vi "Tiepie-Initialize-2018-04-26.vi"(3 "error in (no error)":errorcluster, 4 "Sample Frequency/Hz":i32=500000000, 5 "Record Length/Samples":u64=50000, 6 "TiepieID":i32=33474) -> (0 "error out":errorcluster, 1 "TpDeviceHandle_t":u32, 2 "Card-OK":bool)   [LabVIEW 2013]
panel:
  in  "Channel 1_Range":dbl(ring)=0.4 items=["80 V"=80.0, "40 V"=40.0, "20 V"=20.0, "8 V"=8.0, "4 V"=4.0, "2 V"=2.0, "800 mV"=0.8, "400 mV"=0.4, "200 mV"=0.2]
  in  "CH1_Coupling":u64(ring)=1 items=["Volt DC"=1, "Volt AC"=2, "Ampere DC"=4, "Ampere AC"=8, "Ohm"=16]
  out "channelCount":u16
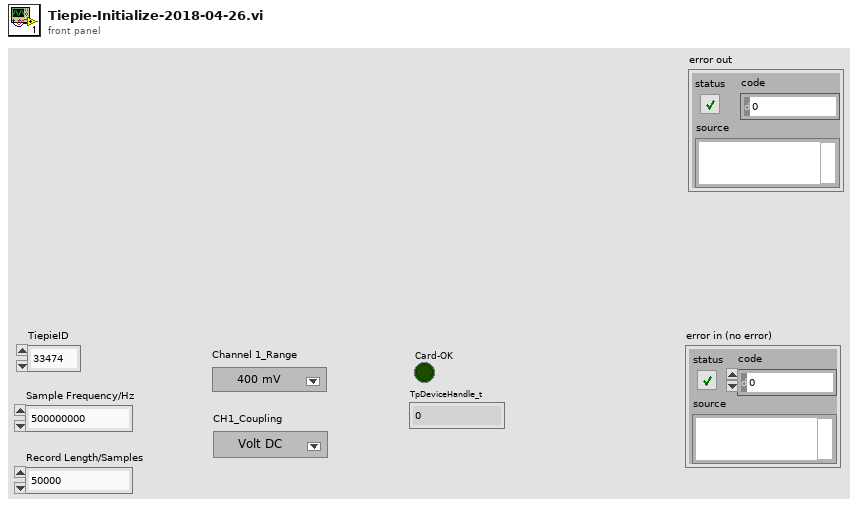
[diagram p1: front panel]
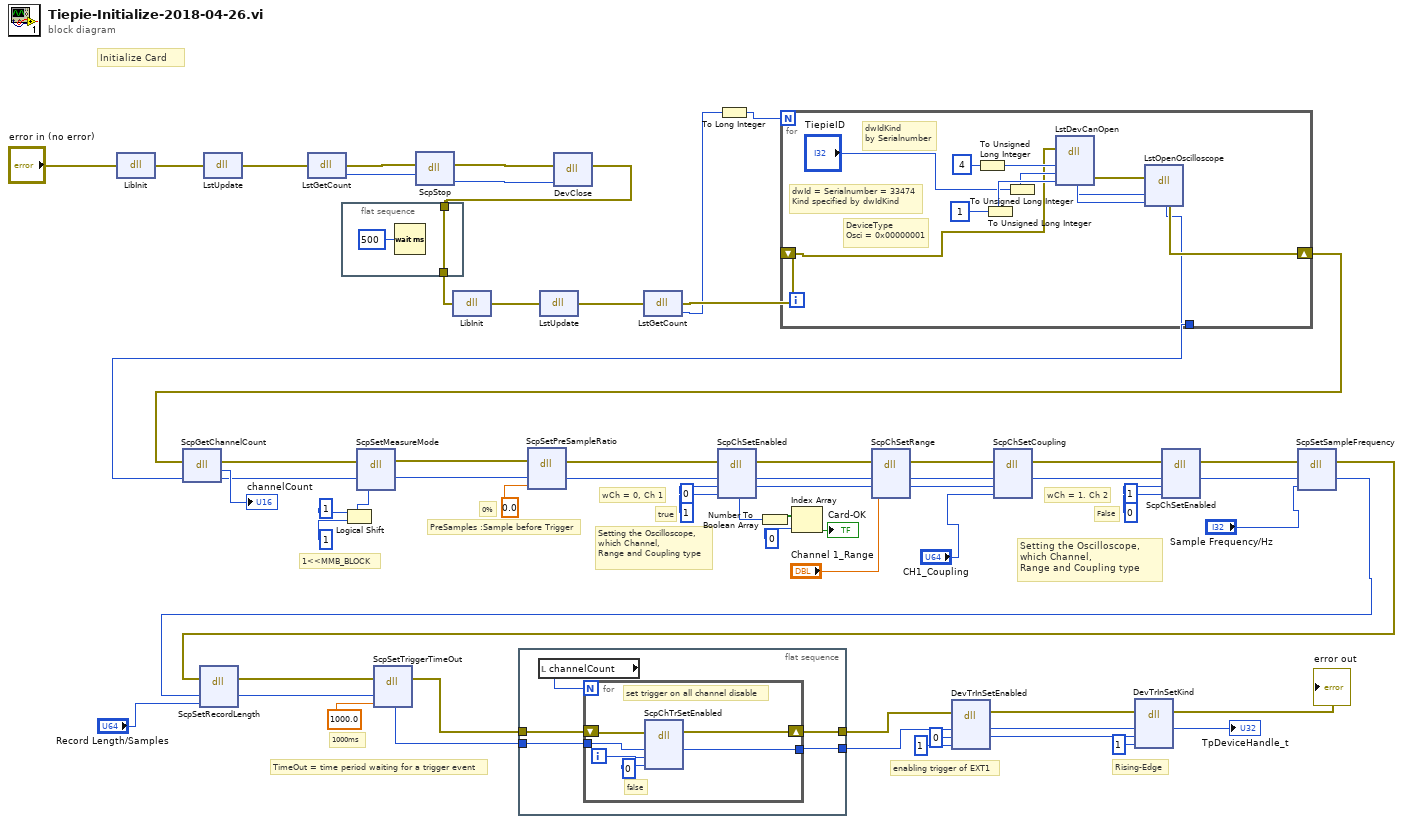
[diagram p0: block diagram]
diagram:
  # "Rising-Edge"
  # "enabling trigger of EXT1"
  # "1000ms"
  # "TimeOut = time period waiting for a trigger event"
  # "Setting the Oscilloscope,\nwhich Channel, \nRange and Coupling type"
  # "wCh = 1. Ch 2"
  # "False"
  # "Setting the Oscilloscope,\nwhich Channel, \nRange and Coupling type"
  # "wCh = 0, Ch 1"
  # "true"
  # "0%"
  # "PreSamples :Sample before Trigger"
  # "1<<MMB_BLOCK"
  # "Initialize Card"
  n1 = dll-call lib="PTH1Labs CUsers82158DesktopSMMSTOF software\t数据卡\nlibtiepie.dll" fn="LibInit"(error in="error in (no error)") -> (error out=w66:errorcluster)  [unwired: 3 in, 1 out]
  n2 = dll-call lib="PTH1Labs CUsers82158DesktopSMMSTOF software\t数据卡\nlibtiepie.dll" fn="LstUpdate"(error in=w66) -> (error out=w23:errorcluster)  [unwired: 3 in, 1 out]
  n3 = dll-call lib="PTH1Labs CUsers82158DesktopSMMSTOF software\t数据卡\nlibtiepie.dll" fn="LstGetCount"(error in=w23) -> (error out=w18:errorcluster, "Count"=w17:u32)  [unwired: 2 in, 1 out]
  n4 = flat-sequence {
    tunnel: w9 -> [w68]
    tunnel: [w68] -> w8
    frame #0 {
      n5 = Wait (ms)(milliseconds to wait=u32 500) -> ()  [unwired: 1 out]
    }
  }
  n6 = Logical Shift(y=u32 1, x=u32 1 ("y")) -> (x << y=w42:u32)
  n7 = dll-call lib="PTH1Labs CUsers82158DesktopSMMSTOF software\t数据卡\nlibtiepie.dll" fn="ScpStop"(error in=w18, "TpDeviceHandle_t"=w17) -> (error out=w16:errorcluster, "TpDeviceHandle_t"=w15:u32)  [unwired: 3 in, 1 out]
  n8 = dll-call lib="PTH1Labs CUsers82158DesktopSMMSTOF software\t数据卡\nlibtiepie.dll" fn="LibInit"(error in=w8) -> (error out=w14:errorcluster)  [unwired: 3 in, 1 out]
  n9 = flat-sequence {
    tunnel: w26 -> [w73]
    tunnel: w27 -> [w72]
    tunnel: [w70] -> w35
    tunnel: [w69] -> w36
    frame #0 {
      n10 = local read "channelCount"() -> (w71:u16)
      n11 = for {
        N: w71 -> [_]
        tunnel: w73 -> [w76]
        shift-right: [w75] -> w70
        shift-left: w72 -> [w77]
        tunnel: [w74] -> w69
        i -> [w79]
        # "set trigger on all channel disable"
        # "false"
        n12 = dll-call lib="PTH1Labs CUsers82158DesktopSMMSTOF software\t数据卡\nlibtiepie.dll" fn="ScpChTrSetEnabled"(error in=w77, "TpDeviceHandle_t"=w76, "wCh"=w79, "bEnable"=u8 0) -> (error out=w75:errorcluster, "TpDeviceHandle_t"=w74:u32)  [unwired: 5 in, 1 out]
      }
    }
  }
  n13 = dll-call lib="PTH1Labs CUsers82158DesktopSMMSTOF software\t数据卡\nlibtiepie.dll" fn="LstUpdate"(error in=w14) -> (error out=w13:errorcluster)  [unwired: 3 in, 1 out]
  n14 = dll-call lib="PTH1Labs CUsers82158DesktopSMMSTOF software\t数据卡\nlibtiepie.dll" fn="DevClose"(error in=w16, "hDevice"=w15) -> (error out=w9:errorcluster)  [unwired: 4 in, 1 out]
  n15 = dll-call lib="PTH1Labs CUsers82158DesktopSMMSTOF software\t数据卡\nlibtiepie.dll" fn="LstGetCount"(error in=w13) -> (error out=w12:errorcluster, "Count"=w11:u32)  [unwired: 2 in, 1 out]
  n16 = To Long Integer(number=w11) -> (32bit integer=w10:i32)
  n17 = for {
    N: w10 -> [_]
    shift-right: [w82] -> w25
    shift-left: w12 -> [w81]
    tunnel: [w80] -> w24
    # "DeviceType\nOsci = 0x00000001"
    # "dwId = Serialnumber = 33474\nKind specified by dwIdKind"
    # "dwIdKind\nby Serialnumber"
    n18 = To Unsigned Long Integer(number=4) -> (unsigned 32bit integer=w90:u32)
    n19 = To Unsigned Long Integer(number=1) -> (unsigned 32bit integer=w88:u32)
    n20 = To Unsigned Long Integer(number="TiepieID") -> (unsigned 32bit integer=w86:u32)
    n21 = dll-call lib="PTH1Labs CUsers82158DesktopSMMSTOF software\t数据卡\nlibtiepie.dll" fn="LstDevCanOpen"(error in=w81, "dwIdKind"=w90, "dwId"=w86, "dwDeviceType"=w88) -> (error out=w83:errorcluster, "dwIdKind"=w84:u32, "dwId"=w85:u32)  [unwired: 4 in, 1 out]
    n22 = dll-call lib="PTH1Labs CUsers82158DesktopSMMSTOF software\t数据卡\nlibtiepie.dll" fn="LstOpenOscilloscope"(error in=w83, "dwIdKind"=w84, "dwId"=w85) -> (error out=w82:errorcluster, "TpDeviceHandle_t"=w80:u32)  [unwired: 4 in, 1 out]
  }
  n23 = dll-call lib="PTH1Labs CUsers82158DesktopSMMSTOF software\t数据卡\nlibtiepie.dll" fn="ScpGetChannelCount"(error in=w25, "TpDeviceHandle_t"=w24) -> (error out=w38:errorcluster, "channelCount"=→"channelCount":u16, "TpDeviceHandle_t"=w37:u32)  [unwired: 2 in, 1 out]
  n24 = dll-call lib="PTH1Labs CUsers82158DesktopSMMSTOF software\t数据卡\nlibtiepie.dll" fn="ScpSetMeasureMode"(error in=w38, "TpDeviceHandle_t"=w37, "dwMeasureMode"=w42) -> (error out=w47:errorcluster, "TpDeviceHandle_t"=w48:u32)  [unwired: 4 in, 1 out]
  n25 = dll-call lib="PTH1Labs CUsers82158DesktopSMMSTOF software\t数据卡\nlibtiepie.dll" fn="ScpSetPreSampleRatio"(error in=w47, "TpDeviceHandle_t"=w48, "dPreSampleRatio"=0.0) -> (error out=w44:errorcluster, "TpDeviceHandle_t"=w46:u32)  [unwired: 4 in, 1 out]
  n26 = dll-call lib="PTH1Labs CUsers82158DesktopSMMSTOF software\t数据卡\nlibtiepie.dll" fn="ScpChSetEnabled"(error in=w44, "TpDeviceHandle_t"=w46, "wCh"=u16 0, "bEnable"=u8 1) -> (error out=w52:errorcluster, "Enabled"=w58:u8, "TpDeviceHandle_t"=w59:u32, "wCh"=w53:u16)  [unwired: 3 in, 1 out]
  n27 = Number To Boolean Array(number=w58) -> (Boolean array=w55:bool[])
  n28 = Index Array(array=w55, index=0) -> (element=→"Card-OK":bool)
  n29 = dll-call lib="PTH1Labs CUsers82158DesktopSMMSTOF software\t数据卡\nlibtiepie.dll" fn="ScpChSetRange"(error in=w52, "TpDeviceHandle_t"=w59, "wCh"=w53, "dRange"="Channel 1_Range") -> (error out=w60:errorcluster, "TpDeviceHandle_t"=w62:u32, "wCh"=w61:u16)  [unwired: 4 in, 1 out]
  n30 = dll-call lib="PTH1Labs CUsers82158DesktopSMMSTOF software\t数据卡\nlibtiepie.dll" fn="DevTrInSetEnabled"(error in=w35, "hDevice"=w36, "wInput"=u16 0, "enable"=u8 1) -> (error out=w32:errorcluster, "hDevice"=w31:u32, "wInput"=w30:u16)  [unwired: 4 in, 1 out]
  n31 = dll-call lib="PTH1Labs CUsers82158DesktopSMMSTOF software\t数据卡\nlibtiepie.dll" fn="ScpChSetCoupling"(error in=w60, "TpDeviceHandle_t"=w62, "wCh"=w61, "qwCoupling"="CH1_Coupling") -> (error out=w45:errorcluster, "TpDeviceHandle_t"=w65:u32)  [unwired: 5 in, 1 out]
  n32 = dll-call lib="PTH1Labs CUsers82158DesktopSMMSTOF software\t数据卡\nlibtiepie.dll" fn="DevTrInSetKind"(error in=w32, "hDevice"=w31, "wInput"=w30, "qwkind"=u64 1) -> (error out=→"error out":errorcluster, "hDevice"=→"TpDeviceHandle_t":u32)  [unwired: 5 in, 1 out]
  n33 = dll-call lib="PTH1Labs CUsers82158DesktopSMMSTOF software\t数据卡\nlibtiepie.dll" fn="ScpChSetEnabled"(error in=w45, "TpDeviceHandle_t"=w65, "wCh"=u16 1, "bEnable"=u8 0) -> (error out=w49:errorcluster, "TpDeviceHandle_t"=w50:u32)  [unwired: 5 in, 1 out]
  n34 = dll-call lib="PTH1Labs CUsers82158DesktopSMMSTOF software\t数据卡\nlibtiepie.dll" fn="ScpSetSampleFrequency"(error in=w49, "TpDeviceHandle_t"=w50, "SampleFrequency"="Sample Frequency/Hz") -> (error out=w20:errorcluster, "TpDeviceHandle_t"=w19:u32)  [unwired: 4 in, 1 out]
  n35 = dll-call lib="PTH1Labs CUsers82158DesktopSMMSTOF software\t数据卡\nlibtiepie.dll" fn="ScpSetRecordLength"(error in=w20, "TpDeviceHandle_t"=w19, "qwRecordLength"="Record Length/Samples") -> (error out=w22:errorcluster, "TpDeviceHandle_t"=w21:u32)  [unwired: 4 in, 1 out]
  n36 = dll-call lib="PTH1Labs CUsers82158DesktopSMMSTOF software\t数据卡\nlibtiepie.dll" fn="ScpSetTriggerTimeOut"(error in=w22, "TpDeviceHandle_t"=w21, "dTimeOut"=1000.0) -> (error out=w27:errorcluster, "TpDeviceHandle_t"=w26:u32)  [unwired: 4 in, 1 out]
